vi "LVFunction_Imop_Compute_PupilRegionsStats.vi"(0 "Pupil.lvclass":refnum<class "Pupil.lvclass">, 11 "error in":errorcluster) -> (4 "Pupil.lvclass":refnum<class "Pupil.lvclass">, 6 "nb_black_regions":i32, 8 "nb_white_regions":i32, 10 "nb_regions":i32, 15 "error out":errorcluster)   [LabVIEW 2020]
doc: "Compute the geometric parameters of the Legendre pupil from a cPupil input.\n\n--------------------------------------------------------------------------------\n\nPupilIn\n cPupil object.\n\nPupilOut\n cPupil object.\n\ncenter\n center coordinates.\n\nsize\n dimensions (width, height) of the square pupil detected\n\nErrorIn\n Error\nErrorOut\n Error"
uses:
  Pupil.lvclass
  LVClass_Pupil Read Pupil.vi
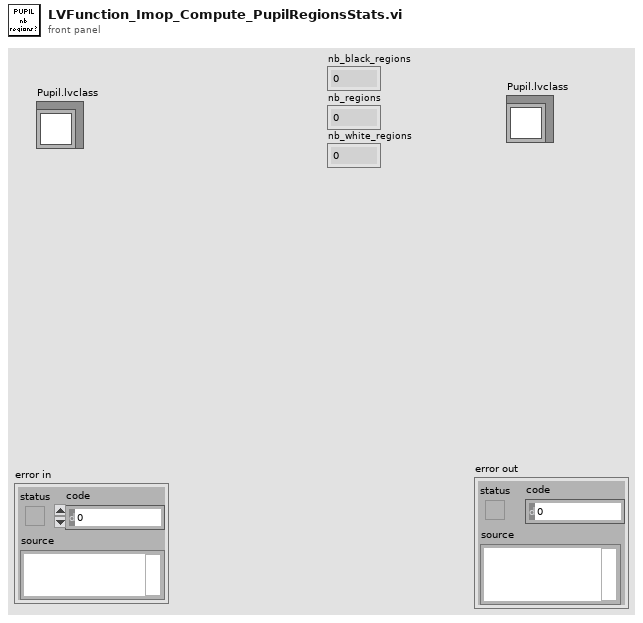
[diagram p1: front panel]
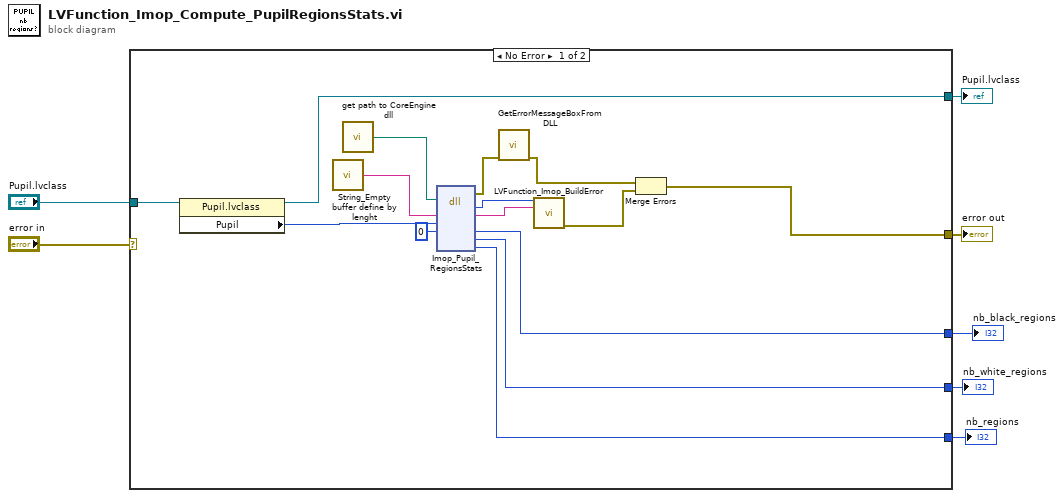
[diagram p0: block diagram]
diagram:
  n1 = case shown="No Error" "error in" {
    selector: "error in" -> [_ w24]
    tunnel: "Pupil.lvclass" -> [w13 w23]
    tunnel: [w21 w24] -> w5
    tunnel: [w12 w23] -> w4
    tunnel: [w10 _] -> w3
    tunnel: [w9 _] -> w2
    tunnel: [w8 _] -> w1
    frame No Error {
      n2 = property class="Pupil.lvclass"(reference=w13) -> (reference out=w12:refnum<class "Pupil.lvclass">, "Pupil"=w22:i32)  [unwired: 1 in, 1 out]
      n3 = call "String_Empty buffer define by lenght.vi"() -> ("Empty buffer"=w20:string)  [unwired: 1 in]
      n4 = call "get path to CoreEngine dll.vi"() -> ("path to c_interface_vc100.dll"=w17:path)  [unwired: 12 in, 3 out]
      n5 = dll-call lib="D:/FLE/0.Code/CoreEngine4_Suite/LV2011_interface/DLLs/c_interface_vc100.dll" fn="Imop_Pupil_RegionsStats"(path in=w17, "message"=w20, "Pupil"=w22, "nb_black_regions"=0) -> (error out=w16:errorcluster, "return type"=w18:i32, "message"=w19:string, "nb_black_regions"=w10:i32, "nb_white_regions"=w8:i32, "nb_regions"=w9:i32)  [unwired: 5 in, 1 out]
      n6 = call "GetErrorMessageBoxFromDLL.vi"("error IN"=w16) -> ("error OUT"=w15:errorcluster)  [unwired: 10 in]
      n7 = call "LVFunction_Imop_BuildError.vi"("code"=w18, "String to Prepend to source (\"\")"=w19) -> ("error out"=w14:errorcluster)  [unwired: 13 in]
      n8 = Merge Errors(w15, w14) -> (w21:errorcluster)
    }
    frame Error {
    }
  }
  "error out" <- w5
  "Pupil.lvclass" <- w4
  "nb_black_regions" <- w3
  "nb_regions" <- w2
  "nb_white_regions" <- w1
